vi "peak - simple guess at omega.vi"(8 "4corners":T1={"z (-pi/2)"=-1.0311345636926572+0.5736824521422934i, "z(inf)"=-0.5200164984937075+1.0975277942502903i, "z (pi/2)"=-1.0311345636926572+0.5736824521422934i, "z center"=-0.5136528600391839+0.580046090596817i, "z(0)"=-0.5200164984937075+1.0975277942502903i, "radius"=-1.0311345636926572}, 10 "omega":dbl[](array[numeric]), 11 "z":cdb[](array[numeric])) -> (1 "guess at gamma":dbl, 2 "guess at omega":dbl)   [LabVIEW 2015]
uses:
  circle corners.ctl
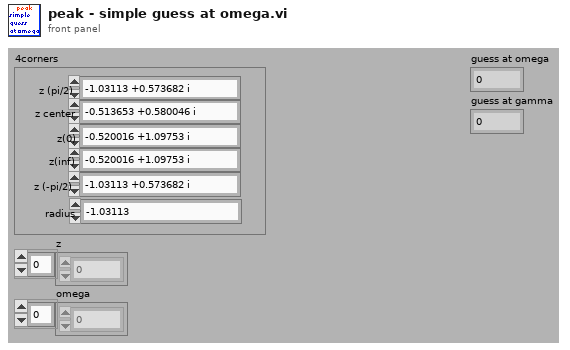
[diagram p1: front panel]
types:
  T1 = typedef "circle corners.ctl" = cluster{"z (-pi/2)":cdb, "z(inf)":cdb, "z (pi/2)":cdb, "z center":cdb, "z(0)":cdb, "radius":dbl}
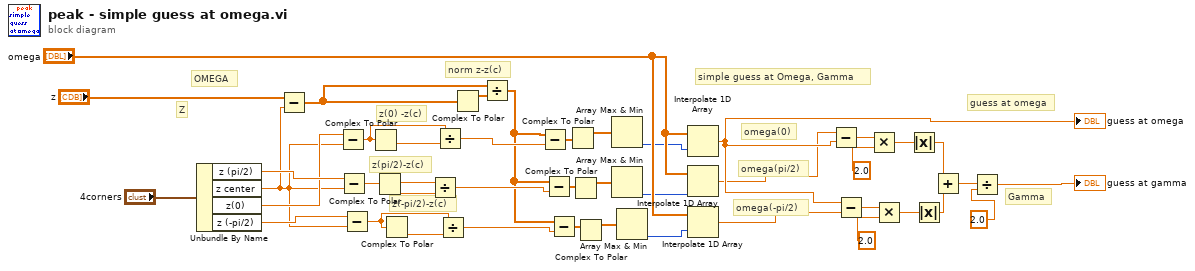
[diagram p0: block diagram]
diagram:
  # "guess at omega"
  # "simple guess at Omega, Gamma"
  # "OMEGA"
  # "Z"
  # "norm z-z(c)"
  # "omega(-pi/2)"
  # "omega(pi/2)"
  # "omega(0)"
  # "Gamma"
  # "z(pi/2)-z(c)"
  # "z(-pi/2)-z(c)"
  # "z(0) -z(c)"
  n1 = Unbundle By Name("4corners") -> ("z (pi/2)"=w37:cdb, "z center"=w4:cdb, "z(0)"=w36:cdb, "z (-pi/2)"=w35:cdb)
  n2 = Subtract(x="z", y=w4) -> (x-y=w2:cdb[])
  n3 = Subtract(x=w36, y=w4) -> (x-y=w34:cdb)
  n4 = Subtract(x=w37, y=w4) -> (x-y=w30:cdb)
  n5 = Subtract(x=w35, y=w4) -> (x-y=w31:cdb)
  n6 = Complex To Polar(r * e^(i*theta)=w34) -> (r=w33:dbl)  [unwired: 1 out]
  n7 = Complex To Polar(r * e^(i*theta)=w30) -> (r=w20:dbl)  [unwired: 1 out]
  n8 = Complex To Polar(r * e^(i*theta)=w31) -> (r=w32:dbl)  [unwired: 1 out]
  n9 = Divide(x=w30, y=w20) -> (x/y=w28:cdb)
  n10 = Divide(x=w34, y=w33) -> (x/y=w29:cdb)
  n11 = Divide(x=w31, y=w32) -> (x/y=w27:cdb)
  n12 = Complex To Polar(r * e^(i*theta)=w2) -> (r=w3:dbl[])  [unwired: 1 out]
  n13 = Divide(x=w2, y=w3) -> (x/y=w1:cdb[])
  n14 = Subtract(x=w1, y=w29) -> (x-y=w26:cdb[])
  n15 = Subtract(x=w1, y=w28) -> (x-y=w24:cdb[])
  n16 = Subtract(x=w1, y=w27) -> (x-y=w25:cdb[])
  n17 = Complex To Polar(r * e^(i*theta)=w26) -> (r=w23:dbl[])  [unwired: 1 out]
  n18 = Complex To Polar(r * e^(i*theta)=w24) -> (r=w22:dbl[])  [unwired: 1 out]
  n19 = Complex To Polar(r * e^(i*theta)=w25) -> (r=w21:dbl[])  [unwired: 1 out]
  n20 = Array Max & Min(array=w23) -> (min index (indices)=w9:i32)  [unwired: 3 out]
  n21 = Array Max & Min(array=w22) -> (min index (indices)=w8:i32)  [unwired: 3 out]
  n22 = Array Max & Min(array=w21) -> (min index (indices)=w7:i32)  [unwired: 3 out]
  n23 = Interpolate 1D Array(1:w9, 2:"omega") -> (0:w39:dbl)
  "guess at omega" <- w39
  n24 = Interpolate 1D Array(1:w8, 2:"omega") -> (0:w6:dbl)
  n25 = Interpolate 1D Array(1:w7, 2:"omega") -> (0:w5:dbl)
  n26 = Subtract(x=w6, y=w39) -> (x-y=w19:dbl)
  n27 = Subtract(x=w39, y=w5) -> (x-y=w16:dbl)
  n28 = Multiply(x=w19, y=2.0) -> (x*y=w17:dbl)
  n29 = Multiply(x=w16, y=2.0) -> (x*y=w14:dbl)
  n30 = Absolute Value(x=w17) -> (abs(x)=w13:dbl)
  n31 = Absolute Value(x=w14) -> (abs(x)=w10:dbl)
  n32 = Add(x=w13, y=w10) -> (x+y=w12:dbl)
  n33 = Divide(x=w12, y=2.0) -> (x/y=→"guess at gamma":dbl)
